vi "inertia.vi"(0 "Inertia":T1=[[1.0, 0.0, 0.0], [0.0, 1.0, 0.0], [0.0, 0.0, 1.0]], 2 "Attributes":T2={"origin"="", "mass"="  <mass value = \"1.00\" />\n"}) -> (4 "sdf out":string="<inertial>\n  <mass value = \"1.00\" />\n  <inertia  \nixx = \"1.00\"  ixy = \"0.00\"  ixz = \"0.00\"  iyx = \"0.00\"  iyy = \"1.00\"  iyz = \"0.00\"  izx = \"0.00\"  izy = \"0.00\"  izz = \"1.00\"  \n/>\n\n")   [LabVIEW 2010]
uses:
  <vilib>/Analysis/Matrix/Datatypes/RealMatrix.ctl
  <vilib>/Analysis/Matrix/NI_Matrix.lvlib
  InertiaAttributes.ctl
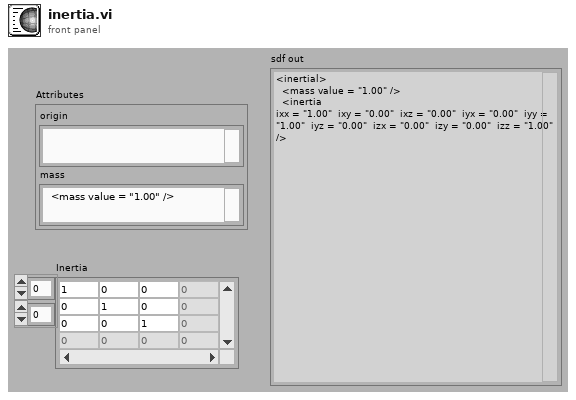
[diagram p1: front panel]
types:
  T1 = typedef "NI_Matrix.lvlib/RealMatrix.ctl" = dbl[][]
  T2 = typedef "InertiaAttributes.ctl" = cluster{"origin":string, "mass":string}
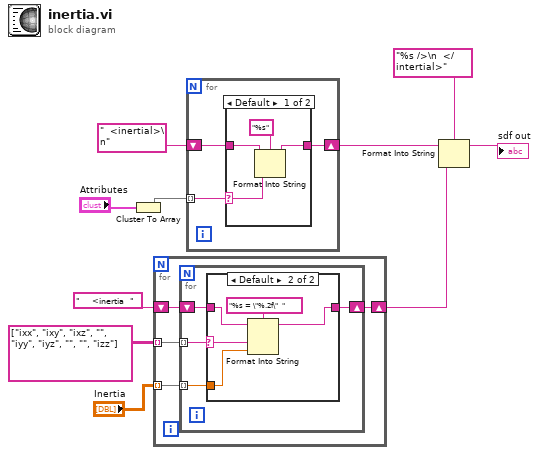
[diagram p0: block diagram]
diagram:
  n1 = Cluster To Array(cluster="Attributes") -> (array=w7:string[])
  n2 = for {
    shift-right: [w11] -> w1
    shift-left: "    <inertia  " -> [w14]
    tunnel: string[][] [["ixx", "ixy", "ixz"], ["", "iyy", "iyz"], ["", "", "izz"]] -> [w13] mode=indexing
    tunnel: "Inertia" -> [w12] mode=indexing
    n3 = for {
      shift-right: [w17] -> w11
      shift-left: w14 -> [w18]
      tunnel: w13 -> [w15] mode=indexing
      tunnel: w12 -> [w16] mode=indexing
      n4 = case shown="Default" w15 {
        selector: w15 -> [_ w20]
        tunnel: w18 -> [w19 w23]
        tunnel: [w19 w22] -> w17
        tunnel: w16 -> [_ w21]
        frame "" {
        }
        frame Default {
          n5 = Format Into String(format string="%s = \"%.2f\"  ", initial string=w23, w20, w21) -> (resulting string=w22:string)  [unwired: 1 in, 1 out]
        }
      }
    }
  }
  n6 = for {
    shift-right: [w27] -> w9
    shift-left: "  <inertial>\n" -> [w26]
    tunnel: w7 -> [w25] mode=indexing
    n7 = case shown="Default" w25 {
      selector: w25 -> [w29 _]
      tunnel: [w28 w32] -> w27
      tunnel: w26 -> [w31 w32]
      frame Default {
        n8 = Format Into String(format string="%s", initial string=w31, w29) -> (resulting string=w28:string)  [unwired: 1 in, 1 out]
      }
      frame "" {
      }
    }
  }
  n9 = Format Into String(format string="%s />\n  </intertial>", initial string=w9, w1) -> (resulting string=→"sdf out":string)  [unwired: 1 in, 1 out]
